vi "S4GUI_003.vi"(7 "Tab ObsEng":enum32{"Obs", "CCD modes", "Guider", "Eng"}(tab)) -> ()   [LabVIEW 2018] (continued)
                n3977 = call-dynamic "Read Channel.vi"("error in (no error)"=w9182, "Acquisition in"=w9181) -> ("error out"=w9184:errorcluster, "Channel.lvclass"=w9183:refnum<class "Channel.lvclass">, "Acquisition out"=w9190:refnum<class "Acquisition.lvclass">)  [unwired: 7 in]
                n3978 = call-dynamic "Read State Machine.vi"("error in (no error)"=w9184, "Device in"=w9183) -> ("error out"=w9186:errorcluster, "State Machine.lvclass"=w9185:refnum<class "State Machine.lvclass">, "Device out"=w9188:refnum<class "Channel.lvclass">)  [unwired: 7 in]
                n3979 = call "Next State.vi"("error in (no error)"=w9186, "New_State"=u32 70, "State Machine in"=w9185) -> ("error out"=w9189:errorcluster, "State Machine out"=w9187:refnum<class "State Machine.lvclass">)  [unwired: 7 in]
                n3980 = call-dynamic "Write State Machine.vi"("error in (no error)"=w9189, "State Machine.lvclass"=w9187, "Device in"=w9188) -> ("error out"=w9191:errorcluster, "Device out"=w9192:refnum<class "Channel.lvclass">)  [unwired: 7 in]
                n3981 = call-dynamic "Write Channel.vi"("error in (no error)"=w9191, "Channel.lvclass"=w9192, "Acquisition in"=w9190) -> ("error out"=w9178:errorcluster, "Acquisition out"=w9179:refnum<class "Acquisition.lvclass">)  [unwired: 7 in]
              }
              frame Enabled {
                # "Não precisa enviar comando STOP para o ACS\nenquanto o controle dos ciclos for feito pela GUI."
              }
            }
            n3982 = call-dynamic "Write Acq_state.vi"("error in (no error)"=w9170, "Acq_state"=u32 0, "Acquisition in"=w9171) -> ("error out"=w9169:errorcluster, "Acquisition out"=w9168:refnum<class "Acquisition.lvclass">)  [unwired: 7 in]
            n3983 = call-dynamic "Write AcquisitionC.vi"("error in (no error)"=w9169, "Acquisition.lvclass"=w9168, "S4ACS_GUI in"=w9174) -> ("error out"=w9156:errorcluster, "S4ACS_GUI out"=w9154:refnum<class "S4GUI.lvclass">)  [unwired: 7 in]
            n3984 = call "Read Instrument.lvclass.vi"("error in (no error)"=w9156, "S4ACS_GUI in"=w9154) -> ("error out"=w9163:errorcluster, "Instrument.lvclass"=w9166:refnum<class "Instrument.lvclass">, "S4ACS_GUI out"=w9167:refnum<class "S4GUI.lvclass">)  [unwired: 7 in]
            n3985 = call "Read WPROT.vi"("error in (no error)"=w9163, "Instrument in"=w9166) -> ("error out"=w9162:errorcluster, "Opt_Selector.lvclass"=w9164:refnum<class "Opt_Selector.lvclass">, "Instrument out"=w9165:refnum<class "Instrument.lvclass">)  [unwired: 7 in]
            n3986 = call-dynamic "Read sequencia_ant.vi"("error in (no error)"=w9162, "Opt_Selector in"=w9164) -> ("error out"=w9158:errorcluster, "sequencia_ant"=w9157:u16, "Opt_Selector out"=w9159:refnum<class "Opt_Selector.lvclass">)  [unwired: 7 in]
            n3987 = call-dynamic "Write sequencia.vi"("error in (no error)"=w9158, "sequencia"=w9157, "Opt_Selector in"=w9159) -> ("error out"=w9145:errorcluster, "Opt_Selector out"=w9148:refnum<class "Opt_Selector.lvclass">)  [unwired: 7 in]
            n3988 = call-dynamic "Read State Machine.vi"("error in (no error)"=w9145, "Device in"=w9148) -> ("error out"=w9150:errorcluster, "State Machine.lvclass"=w9153:refnum<class "State Machine.lvclass">, "Device out"=w9147:refnum<class "Opt_Selector.lvclass">)  [unwired: 7 in]
            n3989 = call "Next State.vi"("error in (no error)"=w9150, "New_State"=10, "State Machine in"=w9153) -> ("error out"=w9149:errorcluster, "State Machine out"=w9152:refnum<class "State Machine.lvclass">)  [unwired: 7 in]
            n3990 = call-dynamic "Write State Machine.vi"("error in (no error)"=w9149, "State Machine.lvclass"=w9152, "Device in"=w9147) -> ("error out"=w9144:errorcluster, "Device out"=w9146:refnum<class "Opt_Selector.lvclass">)  [unwired: 7 in]
            n3991 = call "Write WPROT.vi"("error in (no error)"=w9144, "Opt_Selector.lvclass"=w9146, "Instrument in"=w9165) -> ("error out"=w9161:errorcluster, "Instrument out"=w9160:refnum<class "Instrument.lvclass">)  [unwired: 7 in]
            n3992 = call "Write Instrument.lvclass.vi"("error in (no error)"=w9161, "Instrument.lvclass"=w9160, "S4ACS_GUI in"=w9167) -> ("error out"=w9155:errorcluster, "S4ACS_GUI out"=w9143:refnum<class "S4GUI.lvclass">)  [unwired: 7 in]
          }
          frame Enabled {
            w9200 = FALSE ("Wait Until Done")
            n3993 = call <vilib>:"Application Directory.vi"() -> ("Application Directory"=w9195:path)
            n3994 = Build Path(base path=w9195, name or relative path="MsgStop3.vi") -> (appended path=w9203:path)
            n3995 = Open VI Reference(vi path=w9203, error in (no error)=w9198) -> (vi reference=w9202:refnum<vi>, error out=w9201:errorcluster)  [unwired: 4 in]
            n3996 = invoke class="VI" method="Run VI"(reference=w9202, error in=w9201, "Wait until done"=w9200, "Auto Dispose Ref"=w9200) -> (error out=w9197:errorcluster)  [unwired: 1 in, 4 out]
          }
        }
      }
      event "Stop ch4": Value Change {
        n3997 = event-data() -> ()  [unwired: 1 in, 6 out]
        n3998 = disable-structure shown="Enabled" {
          disable-tunnel: w9207 -> [w9240 w9261]
          disable-tunnel: w9206 -> [w9238 w9263]
          disable-tunnel: [w9220 w9262] -> w9205
          disable-tunnel: [w9208 w9261] -> w9204
          frame Disabled {
            # "Para movimento \nda lamina retardadora"
            # "Restaura a última sequência de lâminas"
            n3999 = call-dynamic "Read AcquisitionD.vi"("error in (no error)"=w9238, "S4ACS_GUI in"=w9240) -> ("error out"=w9242:errorcluster, "Acquisition.lvclass"=w9241:refnum<class "Acquisition.lvclass">, "S4ACS_GUI out"=w9239:refnum<class "S4GUI.lvclass">)  [unwired: 7 in]
            n4000 = disable-structure shown="Enabled" {
              disable-tunnel: w9242 -> [w9247 w9258]
              disable-tunnel: w9241 -> [w9246 w9259]
              disable-tunnel: [w9244 w9259] -> w9236
              disable-tunnel: [w9243 w9258] -> w9235
              frame Disabled {
                # "Só precisa enviar comando STOP quando\no controle dos ciclos for feito pelo ACS."
                n4001 = call-dynamic "Read Channel.vi"("error in (no error)"=w9247, "Acquisition in"=w9246) -> ("error out"=w9249:errorcluster, "Channel.lvclass"=w9248:refnum<class "Channel.lvclass">, "Acquisition out"=w9255:refnum<class "Acquisition.lvclass">)  [unwired: 7 in]
                n4002 = call-dynamic "Read State Machine.vi"("error in (no error)"=w9249, "Device in"=w9248) -> ("error out"=w9251:errorcluster, "State Machine.lvclass"=w9250:refnum<class "State Machine.lvclass">, "Device out"=w9253:refnum<class "Channel.lvclass">)  [unwired: 7 in]
                n4003 = call "Next State.vi"("error in (no error)"=w9251, "New_State"=u32 70, "State Machine in"=w9250) -> ("error out"=w9254:errorcluster, "State Machine out"=w9252:refnum<class "State Machine.lvclass">)  [unwired: 7 in]
                n4004 = call-dynamic "Write State Machine.vi"("error in (no error)"=w9254, "State Machine.lvclass"=w9252, "Device in"=w9253) -> ("error out"=w9256:errorcluster, "Device out"=w9257:refnum<class "Channel.lvclass">)  [unwired: 7 in]
                n4005 = call-dynamic "Write Channel.vi"("error in (no error)"=w9256, "Channel.lvclass"=w9257, "Acquisition in"=w9255) -> ("error out"=w9243:errorcluster, "Acquisition out"=w9244:refnum<class "Acquisition.lvclass">)  [unwired: 7 in]
              }
              frame Enabled {
                # "Não precisa enviar comando STOP para o ACS\nenquanto o controle dos ciclos for feito pela GUI."
              }
            }
            n4006 = call-dynamic "Write Acq_state.vi"("error in (no error)"=w9235, "Acq_state"=u32 0, "Acquisition in"=w9236) -> ("error out"=w9234:errorcluster, "Acquisition out"=w9233:refnum<class "Acquisition.lvclass">)  [unwired: 7 in]
            n4007 = call-dynamic "Write AcquisitionD.vi"("error in (no error)"=w9234, "Acquisition.lvclass"=w9233, "S4ACS_GUI in"=w9239) -> ("error out"=w9221:errorcluster, "S4ACS_GUI out"=w9219:refnum<class "S4GUI.lvclass">)  [unwired: 7 in]
            n4008 = call "Read Instrument.lvclass.vi"("error in (no error)"=w9221, "S4ACS_GUI in"=w9219) -> ("error out"=w9228:errorcluster, "Instrument.lvclass"=w9231:refnum<class "Instrument.lvclass">, "S4ACS_GUI out"=w9232:refnum<class "S4GUI.lvclass">)  [unwired: 7 in]
            n4009 = call "Read WPROT.vi"("error in (no error)"=w9228, "Instrument in"=w9231) -> ("error out"=w9227:errorcluster, "Opt_Selector.lvclass"=w9229:refnum<class "Opt_Selector.lvclass">, "Instrument out"=w9230:refnum<class "Instrument.lvclass">)  [unwired: 7 in]
            n4010 = call-dynamic "Read sequencia_ant.vi"("error in (no error)"=w9227, "Opt_Selector in"=w9229) -> ("error out"=w9223:errorcluster, "sequencia_ant"=w9222:u16, "Opt_Selector out"=w9224:refnum<class "Opt_Selector.lvclass">)  [unwired: 7 in]
            n4011 = call-dynamic "Write sequencia.vi"("error in (no error)"=w9223, "sequencia"=w9222, "Opt_Selector in"=w9224) -> ("error out"=w9210:errorcluster, "Opt_Selector out"=w9213:refnum<class "Opt_Selector.lvclass">)  [unwired: 7 in]
            n4012 = call-dynamic "Read State Machine.vi"("error in (no error)"=w9210, "Device in"=w9213) -> ("error out"=w9215:errorcluster, "State Machine.lvclass"=w9218:refnum<class "State Machine.lvclass">, "Device out"=w9212:refnum<class "Opt_Selector.lvclass">)  [unwired: 7 in]
            n4013 = call "Next State.vi"("error in (no error)"=w9215, "New_State"=10, "State Machine in"=w9218) -> ("error out"=w9214:errorcluster, "State Machine out"=w9217:refnum<class "State Machine.lvclass">)  [unwired: 7 in]
            n4014 = call-dynamic "Write State Machine.vi"("error in (no error)"=w9214, "State Machine.lvclass"=w9217, "Device in"=w9212) -> ("error out"=w9209:errorcluster, "Device out"=w9211:refnum<class "Opt_Selector.lvclass">)  [unwired: 7 in]
            n4015 = call "Write WPROT.vi"("error in (no error)"=w9209, "Opt_Selector.lvclass"=w9211, "Instrument in"=w9230) -> ("error out"=w9226:errorcluster, "Instrument out"=w9225:refnum<class "Instrument.lvclass">)  [unwired: 7 in]
            n4016 = call "Write Instrument.lvclass.vi"("error in (no error)"=w9226, "Instrument.lvclass"=w9225, "S4ACS_GUI in"=w9232) -> ("error out"=w9220:errorcluster, "S4ACS_GUI out"=w9208:refnum<class "S4GUI.lvclass">)  [unwired: 7 in]
          }
          frame Enabled {
            w9265 = FALSE ("Wait Until Done")
            n4017 = call <vilib>:"Application Directory.vi"() -> ("Application Directory"=w9260:path)
            n4018 = Build Path(base path=w9260, name or relative path="MsgStop4.vi") -> (appended path=w9268:path)
            n4019 = Open VI Reference(vi path=w9268, error in (no error)=w9263) -> (vi reference=w9267:refnum<vi>, error out=w9266:errorcluster)  [unwired: 4 in]
            n4020 = invoke class="VI" method="Run VI"(reference=w9267, error in=w9266, "Wait until done"=w9265, "Auto Dispose Ref"=w9265) -> (error out=w9262:errorcluster)  [unwired: 1 in, 4 out]
          }
        }
      }
      event "Pause ch1": Value Change {
        n4021 = event-data() -> ()  [unwired: 1 in, 6 out]
        n4022 = disable-structure shown="Enabled" {
          disable-tunnel: w9272 -> [w9288 w9300]
          disable-tunnel: [w9286 w9298] -> w9271
          disable-tunnel: w9270 -> [w9285 w9299]
          disable-tunnel: [w9273 w9300] -> w9269
          frame Disabled {
            n4023 = call-dynamic "Read AcquisitionA.vi"("error in (no error)"=w9285, "S4ACS_GUI in"=w9288) -> ("error out"=w9280:errorcluster, "Acquisition.lvclass"=w9279:refnum<class "Acquisition.lvclass">, "S4ACS_GUI out"=w9287:refnum<class "S4GUI.lvclass">)  [unwired: 7 in]
            n4024 = call-dynamic "Read Acq_state.vi"("error in (no error)"=w9280, "Acquisition in"=w9279) -> ("error out"=w9282:errorcluster, "Acq_state"=w9283:u32, "Acquisition out"=w9284:refnum<class "Acquisition.lvclass">)  [unwired: 7 in]
            n4025 = call-dynamic "Write Acq_prevstate.vi"("error in (no error)"=w9282, "Acq_prevstate"=w9283, "Acquisition in"=w9284) -> ("error out"=w9277:errorcluster, "Acquisition out"=w9278:refnum<class "Acquisition.lvclass">)  [unwired: 7 in]
            n4026 = call-dynamic "Write Acq_state.vi"("error in (no error)"=w9277, "Acq_state"=u32 400, "Acquisition in"=w9278) -> ("error out"=w9275:errorcluster, "Acquisition out"=w9276:refnum<class "Acquisition.lvclass">)  [unwired: 7 in]
            n4027 = disable-structure shown="Enabled" {
              disable-tunnel: w9275 -> [w9290 w9296]
              disable-tunnel: [w9289 w9296] -> w9274
              frame Disabled {
                n4028 = property on="Start ch1" class="Bool"(error in=w9290, "BoolText.Text"="RESUME" ("Caption.Text")) -> (error out=w9294:errorcluster)  [unwired: 1 in, 1 out]
                n4029 = property on="Pause ch1" class="Bool"(error in=w9294, "DisabledEnum"=T12."Disabled and Grayed Out" ("Disabled")) -> (error out=w9295:errorcluster)  [unwired: 1 in, 1 out]
                n4030 = property on="Start ch1" class="Bool"(error in=w9295, "DisabledEnum"=T12."Enabled" ("Disabled")) -> (error out=w9289:errorcluster)  [unwired: 1 in, 1 out]
              }
              frame Enabled {
              }
            }
            n4031 = call-dynamic "Write AcquisitionA.vi"("error in (no error)"=w9274, "Acquisition.lvclass"=w9276, "S4ACS_GUI in"=w9287) -> ("error out"=w9286:errorcluster, "S4ACS_GUI out"=w9273:refnum<class "S4GUI.lvclass">)  [unwired: 7 in]
          }
          frame Enabled {
            w9302 = FALSE ("Wait Until Done")
            n4032 = call <vilib>:"Application Directory.vi"() -> ("Application Directory"=w9297:path)
            n4033 = Build Path(base path=w9297, name or relative path="MsgPause1.vi") -> (appended path=w9305:path)
            n4034 = Open VI Reference(vi path=w9305, error in (no error)=w9299) -> (vi reference=w9304:refnum<vi>, error out=w9303:errorcluster)  [unwired: 4 in]
            n4035 = invoke class="VI" method="Run VI"(reference=w9304, error in=w9303, "Wait until done"=w9302, "Auto Dispose Ref"=w9302) -> (error out=w9298:errorcluster)  [unwired: 1 in, 4 out]
          }
        }
      }
      event "Pause ch2": Value Change {
        n4036 = event-data() -> ()  [unwired: 1 in, 6 out]
        n4037 = disable-structure shown="Enabled" {
          disable-tunnel: w9309 -> [w9324 w9326]
          disable-tunnel: [w9322 w9327] -> w9308
          disable-tunnel: w9307 -> [w9321 w9328]
          disable-tunnel: [w9311 w9326] -> w9306
          frame Disabled {
            n4038 = call "Read AcquisitionB.vi"("error in (no error)"=w9321, "S4ACS_GUI in"=w9324) -> ("error out"=w9316:errorcluster, "Acquisition.lvclass"=w9315:refnum<class "Acquisition.lvclass">, "S4ACS_GUI out"=w9323:refnum<class "S4GUI.lvclass">)  [unwired: 7 in]
            n4039 = call-dynamic "Read Acq_state.vi"("error in (no error)"=w9316, "Acquisition in"=w9315) -> ("error out"=w9318:errorcluster, "Acq_state"=w9319:u32, "Acquisition out"=w9320:refnum<class "Acquisition.lvclass">)  [unwired: 7 in]
            n4040 = call-dynamic "Write Acq_prevstate.vi"("error in (no error)"=w9318, "Acq_prevstate"=w9319, "Acquisition in"=w9320) -> ("error out"=w9313:errorcluster, "Acquisition out"=w9314:refnum<class "Acquisition.lvclass">)  [unwired: 7 in]
            n4041 = call-dynamic "Write Acq_state.vi"("error in (no error)"=w9313, "Acq_state"=u32 400, "Acquisition in"=w9314) -> ("error out"=w9310:errorcluster, "Acquisition out"=w9312:refnum<class "Acquisition.lvclass">)  [unwired: 7 in]
            n4042 = call "Write AcquisitionB.vi"("error in (no error)"=w9310, "Acquisition.lvclass"=w9312, "S4ACS_GUI in"=w9323) -> ("error out"=w9322:errorcluster, "S4ACS_GUI out"=w9311:refnum<class "S4GUI.lvclass">)  [unwired: 7 in]
          }
          frame Enabled {
            w9330 = FALSE ("Wait Until Done")
            n4043 = call <vilib>:"Application Directory.vi"() -> ("Application Directory"=w9325:path)
            n4044 = Build Path(base path=w9325, name or relative path="MsgPause2.vi") -> (appended path=w9333:path)
            n4045 = Open VI Reference(vi path=w9333, error in (no error)=w9328) -> (vi reference=w9332:refnum<vi>, error out=w9331:errorcluster)  [unwired: 4 in]
            n4046 = invoke class="VI" method="Run VI"(reference=w9332, error in=w9331, "Wait until done"=w9330, "Auto Dispose Ref"=w9330) -> (error out=w9327:errorcluster)  [unwired: 1 in, 4 out]
          }
        }
      }
      event "Pause ch3": Value Change {
        n4047 = event-data() -> ()  [unwired: 1 in, 6 out]
        n4048 = disable-structure shown="Enabled" {
          disable-tunnel: w9337 -> [w9352 w9354]
          disable-tunnel: [w9350 w9355] -> w9336
          disable-tunnel: w9335 -> [w9349 w9356]
          disable-tunnel: [w9339 w9354] -> w9334
          frame Disabled {
            n4049 = call-dynamic "Read AcquisitionC.vi"("error in (no error)"=w9349, "S4ACS_GUI in"=w9352) -> ("error out"=w9344:errorcluster, "Acquisition.lvclass"=w9343:refnum<class "Acquisition.lvclass">, "S4ACS_GUI out"=w9351:refnum<class "S4GUI.lvclass">)  [unwired: 7 in]
            n4050 = call-dynamic "Read Acq_state.vi"("error in (no error)"=w9344, "Acquisition in"=w9343) -> ("error out"=w9346:errorcluster, "Acq_state"=w9347:u32, "Acquisition out"=w9348:refnum<class "Acquisition.lvclass">)  [unwired: 7 in]
            n4051 = call-dynamic "Write Acq_prevstate.vi"("error in (no error)"=w9346, "Acq_prevstate"=w9347, "Acquisition in"=w9348) -> ("error out"=w9341:errorcluster, "Acquisition out"=w9342:refnum<class "Acquisition.lvclass">)  [unwired: 7 in]
            n4052 = call-dynamic "Write Acq_state.vi"("error in (no error)"=w9341, "Acq_state"=u32 400, "Acquisition in"=w9342) -> ("error out"=w9338:errorcluster, "Acquisition out"=w9340:refnum<class "Acquisition.lvclass">)  [unwired: 7 in]
            n4053 = call-dynamic "Write AcquisitionC.vi"("error in (no error)"=w9338, "Acquisition.lvclass"=w9340, "S4ACS_GUI in"=w9351) -> ("error out"=w9350:errorcluster, "S4ACS_GUI out"=w9339:refnum<class "S4GUI.lvclass">)  [unwired: 7 in]
          }
          frame Enabled {
            w9358 = FALSE ("Wait Until Done")
            n4054 = call <vilib>:"Application Directory.vi"() -> ("Application Directory"=w9353:path)
            n4055 = Build Path(base path=w9353, name or relative path="MsgPause3.vi") -> (appended path=w9361:path)
            n4056 = Open VI Reference(vi path=w9361, error in (no error)=w9356) -> (vi reference=w9360:refnum<vi>, error out=w9359:errorcluster)  [unwired: 4 in]
            n4057 = invoke class="VI" method="Run VI"(reference=w9360, error in=w9359, "Wait until done"=w9358, "Auto Dispose Ref"=w9358) -> (error out=w9355:errorcluster)  [unwired: 1 in, 4 out]
          }
        }
      }
      event "Pause ch4": Value Change {
        n4058 = event-data() -> ()  [unwired: 1 in, 6 out]
        n4059 = disable-structure shown="Enabled" {
          disable-tunnel: w9365 -> [w9380 w9389]
          disable-tunnel: [w9378 w9382] -> w9364
          disable-tunnel: w9363 -> [w9377 w9383]
          disable-tunnel: [w9367 w9389] -> w9362
          frame Disabled {
            n4060 = call-dynamic "Read AcquisitionD.vi"("error in (no error)"=w9377, "S4ACS_GUI in"=w9380) -> ("error out"=w9372:errorcluster, "Acquisition.lvclass"=w9371:refnum<class "Acquisition.lvclass">, "S4ACS_GUI out"=w9379:refnum<class "S4GUI.lvclass">)  [unwired: 7 in]
            n4061 = call-dynamic "Read Acq_state.vi"("error in (no error)"=w9372, "Acquisition in"=w9371) -> ("error out"=w9374:errorcluster, "Acq_state"=w9375:u32, "Acquisition out"=w9376:refnum<class "Acquisition.lvclass">)  [unwired: 7 in]
            n4062 = call-dynamic "Write Acq_prevstate.vi"("error in (no error)"=w9374, "Acq_prevstate"=w9375, "Acquisition in"=w9376) -> ("error out"=w9369:errorcluster, "Acquisition out"=w9370:refnum<class "Acquisition.lvclass">)  [unwired: 7 in]
            n4063 = call-dynamic "Write Acq_state.vi"("error in (no error)"=w9369, "Acq_state"=u32 400, "Acquisition in"=w9370) -> ("error out"=w9366:errorcluster, "Acquisition out"=w9368:refnum<class "Acquisition.lvclass">)  [unwired: 7 in]
            n4064 = call-dynamic "Write AcquisitionD.vi"("error in (no error)"=w9366, "Acquisition.lvclass"=w9368, "S4ACS_GUI in"=w9379) -> ("error out"=w9378:errorcluster, "S4ACS_GUI out"=w9367:refnum<class "S4GUI.lvclass">)  [unwired: 7 in]
          }
          frame Enabled {
            w9385 = FALSE ("Wait Until Done")
            n4065 = call <vilib>:"Application Directory.vi"() -> ("Application Directory"=w9381:path)
            n4066 = Build Path(base path=w9381, name or relative path="MsgPause4.vi") -> (appended path=w9388:path)
            n4067 = Open VI Reference(vi path=w9388, error in (no error)=w9383) -> (vi reference=w9387:refnum<vi>, error out=w9386:errorcluster)  [unwired: 4 in]
            n4068 = invoke class="VI" method="Run VI"(reference=w9387, error in=w9386, "Wait until done"=w9385, "Auto Dispose Ref"=w9385) -> (error out=w9382:errorcluster)  [unwired: 1 in, 4 out]
          }
        }
      }
      event "Stop SM": Value Change {
        w9395 = 0.0 ("Scale.Range:Minor Increment")
        n4069 = event-data() -> ()  [unwired: 1 in, 6 out]
        n4070 = call-dynamic "Write User Event.vi"("error in (no error)"=w9393, "User Event"="STOP SM CLICKED", "S4GUI in"=w9394) -> ("error out"=w9391:errorcluster, "S4GUI out"=w9392:refnum<class "S4GUI.lvclass">)  [unwired: 7 in]
        n4071 = disable-structure shown="Enabled" {
          disable-tunnel: w9392 -> [w9432 w9456]
          disable-tunnel: w9391 -> [w9430 w9457]
          disable-tunnel: [w9417 w9455] -> w9397
          disable-tunnel: [w9401 w9456] -> w9396
          frame Disabled {
            # "Não precisa enviar comando STOP para o ACS\nenquanto o controle dos ciclos for feito pela GUI."
            # "Para movimento \nda lamina retardadora"
            # "Restaura a sequencia anterior"
            n4072 = call-dynamic "Read AcquisitionA.vi"("error in (no error)"=w9430, "S4ACS_GUI in"=w9432) -> ("error out"=w9434:errorcluster, "Acquisition.lvclass"=w9433:refnum<class "Acquisition.lvclass">, "S4ACS_GUI out"=w9431:refnum<class "S4GUI.lvclass">)  [unwired: 7 in]
            n4073 = disable-structure shown="Enabled" {
              disable-tunnel: [w9448 w9452] -> w9436
              disable-tunnel: [w9447 w9453] -> w9435
              disable-tunnel: w9434 -> [w9439 w9452]
              disable-tunnel: w9433 -> [w9438 w9453]
              frame Disabled {
                n4074 = call-dynamic "Read Channel.vi"("error in (no error)"=w9439, "Acquisition in"=w9438) -> ("error out"=w9441:errorcluster, "Channel.lvclass"=w9440:refnum<class "Channel.lvclass">, "Acquisition out"=w9449:refnum<class "Acquisition.lvclass">)  [unwired: 7 in]
                n4075 = call-dynamic "Read State Machine.vi"("error in (no error)"=w9441, "Device in"=w9440) -> ("error out"=w9443:errorcluster, "State Machine.lvclass"=w9442:refnum<class "State Machine.lvclass">, "Device out"=w9445:refnum<class "Channel.lvclass">)  [unwired: 7 in]
                n4076 = call "Next State.vi"("error in (no error)"=w9443, "New_State"=u32 70, "State Machine in"=w9442) -> ("error out"=w9446:errorcluster, "State Machine out"=w9444:refnum<class "State Machine.lvclass">)  [unwired: 7 in]
                n4077 = call-dynamic "Write State Machine.vi"("error in (no error)"=w9446, "State Machine.lvclass"=w9444, "Device in"=w9445) -> ("error out"=w9450:errorcluster, "Device out"=w9451:refnum<class "Channel.lvclass">)  [unwired: 7 in]
                n4078 = call-dynamic "Write Channel.vi"("error in (no error)"=w9450, "Channel.lvclass"=w9451, "Acquisition in"=w9449) -> ("error out"=w9448:errorcluster, "Acquisition out"=w9447:refnum<class "Acquisition.lvclass">)  [unwired: 7 in]
              }
              frame Enabled {
              }
            }
            n4079 = call-dynamic "Write AcquisitionA.vi"("error in (no error)"=w9436, "Acquisition.lvclass"=w9435, "S4ACS_GUI in"=w9431) -> ("error out"=w9399:errorcluster, "S4ACS_GUI out"=w9400:refnum<class "S4GUI.lvclass">)  [unwired: 7 in]
            n4080 = call-dynamic "Write Obs_state.vi"("error in (no error)"=w9399, "Obs_state"=u32 0, "S4ACS_GUI in"=w9400) -> ("error out"=w9419:errorcluster, "S4ACS_GUI out"=w9420:refnum<class "S4GUI.lvclass">)  [unwired: 7 in]
            n4081 = call "Read Instrument.lvclass.vi"("error in (no error)"=w9419, "S4ACS_GUI in"=w9420) -> ("error out"=w9428:errorcluster, "Instrument.lvclass"=w9426:refnum<class "Instrument.lvclass">, "S4ACS_GUI out"=w9427:refnum<class "S4GUI.lvclass">)  [unwired: 7 in]
            n4082 = call "Read WPROT.vi"("error in (no error)"=w9428, "Instrument in"=w9426) -> ("error out"=w9413:errorcluster, "Opt_Selector.lvclass"=w9416:refnum<class "Opt_Selector.lvclass">, "Instrument out"=w9425:refnum<class "Instrument.lvclass">)  [unwired: 7 in]
            n4083 = call-dynamic "Read sequencia_ant.vi"("error in (no error)"=w9413, "Opt_Selector in"=w9416) -> ("error out"=w9412:errorcluster, "sequencia_ant"=w9414:u16, "Opt_Selector out"=w9415:refnum<class "Opt_Selector.lvclass">)  [unwired: 7 in]
            n4084 = call-dynamic "Write sequencia.vi"("error in (no error)"=w9412, "sequencia"=w9414, "Opt_Selector in"=w9415) -> ("error out"=w9410:errorcluster, "Opt_Selector out"=w9411:refnum<class "Opt_Selector.lvclass">)  [unwired: 7 in]
            n4085 = call-dynamic "Read State Machine.vi"("error in (no error)"=w9410, "Device in"=w9411) -> ("error out"=w9405:errorcluster, "State Machine.lvclass"=w9408:refnum<class "State Machine.lvclass">, "Device out"=w9409:refnum<class "Opt_Selector.lvclass">)  [unwired: 7 in]
            n4086 = call "Next State.vi"("error in (no error)"=w9405, "New_State"=10, "State Machine in"=w9408) -> ("error out"=w9404:errorcluster, "State Machine out"=w9407:refnum<class "State Machine.lvclass">)  [unwired: 7 in]
            n4087 = call-dynamic "Write State Machine.vi"("error in (no error)"=w9404, "State Machine.lvclass"=w9407, "Device in"=w9409) -> ("error out"=w9403:errorcluster, "Device out"=w9402:refnum<class "Opt_Selector.lvclass">)  [unwired: 7 in]
            n4088 = call "Write WPROT.vi"("error in (no error)"=w9403, "Opt_Selector.lvclass"=w9402, "Instrument in"=w9425) -> ("error out"=w9423:errorcluster, "Instrument out"=w9424:refnum<class "Instrument.lvclass">)  [unwired: 7 in]
            n4089 = call "Write Instrument.lvclass.vi"("error in (no error)"=w9423, "Instrument.lvclass"=w9424, "S4ACS_GUI in"=w9427) -> ("error out"=w9422:errorcluster, "S4ACS_GUI out"=w9421:refnum<class "S4GUI.lvclass">)  [unwired: 7 in]
            n4090 = call-dynamic "Write ciclos.vi"("error in (no error)"=w9422, "ciclos"=u32 0, "S4ACS_GUI in"=w9421) -> ("error out"=w9417:errorcluster, "S4ACS_GUI out"=w9401:refnum<class "S4GUI.lvclass">)  [unwired: 7 in]
          }
          frame Enabled {
            w9459 = FALSE ("Wait Until Done")
            n4091 = call <vilib>:"Application Directory.vi"() -> ("Application Directory"=w9454:path)
            n4092 = Build Path(base path=w9454, name or relative path="MsgStopSync.vi") -> (appended path=w9462:path)
            n4093 = Open VI Reference(vi path=w9462, error in (no error)=w9457) -> (vi reference=w9461:refnum<vi>, error out=w9460:errorcluster)  [unwired: 4 in]
            n4094 = invoke class="VI" method="Run VI"(reference=w9461, error in=w9460, "Wait until done"=w9459, "Auto Dispose Ref"=w9459) -> (error out=w9455:errorcluster)  [unwired: 1 in, 4 out]
          }
        }
        n4095 = property on="#Cycles Done" class="Slide (strict)"(error in=w9397, "Scale.Maximum"=w9395, "Scale.Minimum"=w9395) -> (error out=w9398:errorcluster)  [unwired: 1 in, 1 out]
      }
      event "Abort SM": Value Change {
        w9470 = 0.0 ("Scale.Range:Minor Increment")
        n4096 = event-data() -> ()  [unwired: 1 in, 6 out]
        n4097 = call-dynamic "Write User Event.vi"("error in (no error)"=w9466, "User Event"="ABORT SM CLICKED", "S4GUI in"=w9467) -> ("error out"=w9464:errorcluster, "S4GUI out"=w9465:refnum<class "S4GUI.lvclass">)  [unwired: 7 in]
        n4098 = disable-structure shown="Enabled" {
          disable-tunnel: w9465 -> [w9561 w9585]
          disable-tunnel: w9464 -> [w9559 w9587]
          disable-tunnel: [w9473 w9585] -> w9469
          disable-tunnel: [w9472 w9586] -> w9468
          frame Disabled {
            # "Restaura a sequencia anterior"
            # "Para movimento \nda lamina retardadora"
            n4099 = call-dynamic "Read AcquisitionA.vi"("error in (no error)"=w9559, "S4ACS_GUI in"=w9561) -> ("error out"=w9564:errorcluster, "Acquisition.lvclass"=w9563:refnum<class "Acquisition.lvclass">, "S4ACS_GUI out"=w9560:refnum<class "S4GUI.lvclass">)  [unwired: 7 in]
            n4100 = call-dynamic "Read Channel.vi"("error in (no error)"=w9564, "Acquisition in"=w9563) -> ("error out"=w9566:errorcluster, "Channel.lvclass"=w9565:refnum<class "Channel.lvclass">, "Acquisition out"=w9574:refnum<class "Acquisition.lvclass">)  [unwired: 7 in]
            n4101 = call-dynamic "Read State Machine.vi"("error in (no error)"=w9566, "Device in"=w9565) -> ("error out"=w9568:errorcluster, "State Machine.lvclass"=w9567:refnum<class "State Machine.lvclass">, "Device out"=w9570:refnum<class "Channel.lvclass">)  [unwired: 7 in]
            n4102 = call "Next State.vi"("error in (no error)"=w9568, "New_State"=u32 80, "State Machine in"=w9567) -> ("error out"=w9571:errorcluster, "State Machine out"=w9569:refnum<class "State Machine.lvclass">)  [unwired: 7 in]
            n4103 = call-dynamic "Write State Machine.vi"("error in (no error)"=w9571, "State Machine.lvclass"=w9569, "Device in"=w9570) -> ("error out"=w9575:errorcluster, "Device out"=w9576:refnum<class "Channel.lvclass">)  [unwired: 7 in]
            n4104 = call-dynamic "Write Channel.vi"("error in (no error)"=w9575, "Channel.lvclass"=w9576, "Acquisition in"=w9574) -> ("error out"=w9573:errorcluster, "Acquisition out"=w9572:refnum<class "Acquisition.lvclass">)  [unwired: 7 in]
            n4105 = call-dynamic "Write AcquisitionA.vi"("error in (no error)"=w9573, "Acquisition.lvclass"=w9572, "S4ACS_GUI in"=w9560) -> ("error out"=w9545:errorcluster, "S4ACS_GUI out"=w9544:refnum<class "S4GUI.lvclass">)  [unwired: 7 in]
            n4106 = call "Read AcquisitionB.vi"("error in (no error)"=w9545, "S4ACS_GUI in"=w9544) -> ("error out"=w9538:errorcluster, "Acquisition.lvclass"=w9542:refnum<class "Acquisition.lvclass">, "S4ACS_GUI out"=w9543:refnum<class "S4GUI.lvclass">)  [unwired: 7 in]
            n4107 = call-dynamic "Read Channel.vi"("error in (no error)"=w9538, "Acquisition in"=w9542) -> ("error out"=w9553:errorcluster, "Channel.lvclass"=w9554:refnum<class "Channel.lvclass">, "Acquisition out"=w9540:refnum<class "Acquisition.lvclass">)  [unwired: 7 in]
            n4108 = call-dynamic "Read State Machine.vi"("error in (no error)"=w9553, "Device in"=w9554) -> ("error out"=w9551:errorcluster, "State Machine.lvclass"=w9552:refnum<class "State Machine.lvclass">, "Device out"=w9549:refnum<class "Channel.lvclass">)  [unwired: 7 in]
            n4109 = call "Next State.vi"("error in (no error)"=w9551, "New_State"=u32 80, "State Machine in"=w9552) -> ("error out"=w9548:errorcluster, "State Machine out"=w9550:refnum<class "State Machine.lvclass">)  [unwired: 7 in]
            n4110 = call-dynamic "Write State Machine.vi"("error in (no error)"=w9548, "State Machine.lvclass"=w9550, "Device in"=w9549) -> ("error out"=w9547:errorcluster, "Device out"=w9546:refnum<class "Channel.lvclass">)  [unwired: 7 in]
            n4111 = call-dynamic "Write Channel.vi"("error in (no error)"=w9547, "Channel.lvclass"=w9546, "Acquisition in"=w9540) -> ("error out"=w9539:errorcluster, "Acquisition out"=w9541:refnum<class "Acquisition.lvclass">)  [unwired: 7 in]
            n4112 = call "Write AcquisitionB.vi"("error in (no error)"=w9539, "Acquisition.lvclass"=w9541, "S4ACS_GUI in"=w9543) -> ("error out"=w9505:errorcluster, "S4ACS_GUI out"=w9504:refnum<class "S4GUI.lvclass">)  [unwired: 7 in]
            n4113 = call-dynamic "Read AcquisitionC.vi"("error in (no error)"=w9505, "S4ACS_GUI in"=w9504) -> ("error out"=w9522:errorcluster, "Acquisition.lvclass"=w9526:refnum<class "Acquisition.lvclass">, "S4ACS_GUI out"=w9527:refnum<class "S4GUI.lvclass">)  [unwired: 7 in]
            n4114 = call-dynamic "Read Channel.vi"("error in (no error)"=w9522, "Acquisition in"=w9526) -> ("error out"=w9535:errorcluster, "Channel.lvclass"=w9536:refnum<class "Channel.lvclass">, "Acquisition out"=w9524:refnum<class "Acquisition.lvclass">)  [unwired: 7 in]
            n4115 = call-dynamic "Read State Machine.vi"("error in (no error)"=w9535, "Device in"=w9536) -> ("error out"=w9533:errorcluster, "State Machine.lvclass"=w9534:refnum<class "State Machine.lvclass">, "Device out"=w9531:refnum<class "Channel.lvclass">)  [unwired: 7 in]
            n4116 = call "Next State.vi"("error in (no error)"=w9533, "New_State"=u32 80, "State Machine in"=w9534) -> ("error out"=w9530:errorcluster, "State Machine out"=w9532:refnum<class "State Machine.lvclass">)  [unwired: 7 in]
            n4117 = call-dynamic "Write State Machine.vi"("error in (no error)"=w9530, "State Machine.lvclass"=w9532, "Device in"=w9531) -> ("error out"=w9529:errorcluster, "Device out"=w9528:refnum<class "Channel.lvclass">)  [unwired: 7 in]
            n4118 = call-dynamic "Write Channel.vi"("error in (no error)"=w9529, "Channel.lvclass"=w9528, "Acquisition in"=w9524) -> ("error out"=w9523:errorcluster, "Acquisition out"=w9525:refnum<class "Acquisition.lvclass">)  [unwired: 7 in]
            n4119 = call-dynamic "Write AcquisitionC.vi"("error in (no error)"=w9523, "Acquisition.lvclass"=w9525, "S4ACS_GUI in"=w9527) -> ("error out"=w9503:errorcluster, "S4ACS_GUI out"=w9502:refnum<class "S4GUI.lvclass">)  [unwired: 7 in]
            n4120 = call-dynamic "Read AcquisitionD.vi"("error in (no error)"=w9503, "S4ACS_GUI in"=w9502) -> ("error out"=w9506:errorcluster, "Acquisition.lvclass"=w9510:refnum<class "Acquisition.lvclass">, "S4ACS_GUI out"=w9511:refnum<class "S4GUI.lvclass">)  [unwired: 7 in]
            n4121 = call-dynamic "Read Channel.vi"("error in (no error)"=w9506, "Acquisition in"=w9510) -> ("error out"=w9519:errorcluster, "Channel.lvclass"=w9520:refnum<class "Channel.lvclass">, "Acquisition out"=w9508:refnum<class "Acquisition.lvclass">)  [unwired: 7 in]
            n4122 = call-dynamic "Read State Machine.vi"("error in (no error)"=w9519, "Device in"=w9520) -> ("error out"=w9517:errorcluster, "State Machine.lvclass"=w9518:refnum<class "State Machine.lvclass">, "Device out"=w9515:refnum<class "Channel.lvclass">)  [unwired: 7 in]
            n4123 = call "Next State.vi"("error in (no error)"=w9517, "New_State"=u32 80, "State Machine in"=w9518) -> ("error out"=w9514:errorcluster, "State Machine out"=w9516:refnum<class "State Machine.lvclass">)  [unwired: 7 in]
            n4124 = call-dynamic "Write State Machine.vi"("error in (no error)"=w9514, "State Machine.lvclass"=w9516, "Device in"=w9515) -> ("error out"=w9513:errorcluster, "Device out"=w9512:refnum<class "Channel.lvclass">)  [unwired: 7 in]
            n4125 = call-dynamic "Write Channel.vi"("error in (no error)"=w9513, "Channel.lvclass"=w9512, "Acquisition in"=w9508) -> ("error out"=w9507:errorcluster, "Acquisition out"=w9509:refnum<class "Acquisition.lvclass">)  [unwired: 7 in]
            n4126 = call-dynamic "Write AcquisitionD.vi"("error in (no error)"=w9507, "Acquisition.lvclass"=w9509, "S4ACS_GUI in"=w9511) -> ("error out"=w9500:errorcluster, "S4ACS_GUI out"=w9501:refnum<class "S4GUI.lvclass">)  [unwired: 7 in]
            n4127 = disable-structure shown="Enabled" {
              disable-tunnel: w9501 -> [w9581 w9583]
              disable-tunnel: w9500 -> [w9580 w9582]
              disable-tunnel: [w9578 w9583] -> w9557
              disable-tunnel: [w9577 w9582] -> w9556
              frame Disabled {
                n4128 = call-dynamic "Write aborted.vi"("error in (no error)"=w9580, "aborted"=TRUE ("stopped"), "S4ACS_GUI in"=w9581) -> ("error out"=w9577:errorcluster, "S4ACS_GUI out"=w9578:refnum<class "S4GUI.lvclass">)  [unwired: 7 in]
              }
              frame Enabled {
              }
            }
            n4129 = call-dynamic "Write Obs_state.vi"("error in (no error)"=w9556, "Obs_state"=u32 0, "S4ACS_GUI in"=w9557) -> ("error out"=w9474:errorcluster, "S4ACS_GUI out"=w9475:refnum<class "S4GUI.lvclass">)  [unwired: 7 in]
            n4130 = call "Read Instrument.lvclass.vi"("error in (no error)"=w9474, "S4ACS_GUI in"=w9475) -> ("error out"=w9494:errorcluster, "Instrument.lvclass"=w9496:refnum<class "Instrument.lvclass">, "S4ACS_GUI out"=w9495:refnum<class "S4GUI.lvclass">)  [unwired: 7 in]
            n4131 = call "Read WPROT.vi"("error in (no error)"=w9494, "Instrument in"=w9496) -> ("error out"=w9489:errorcluster, "Opt_Selector.lvclass"=w9492:refnum<class "Opt_Selector.lvclass">, "Instrument out"=w9497:refnum<class "Instrument.lvclass">)  [unwired: 7 in]
            n4132 = call-dynamic "Read sequencia_ant.vi"("error in (no error)"=w9489, "Opt_Selector in"=w9492) -> ("error out"=w9488:errorcluster, "sequencia_ant"=w9490:u16, "Opt_Selector out"=w9491:refnum<class "Opt_Selector.lvclass">)  [unwired: 7 in]
            n4133 = call-dynamic "Write sequencia.vi"("error in (no error)"=w9488, "sequencia"=w9490, "Opt_Selector in"=w9491) -> ("error out"=w9483:errorcluster, "Opt_Selector out"=w9484:refnum<class "Opt_Selector.lvclass">)  [unwired: 7 in]
            n4134 = call-dynamic "Read State Machine.vi"("error in (no error)"=w9483, "Device in"=w9484) -> ("error out"=w9486:errorcluster, "State Machine.lvclass"=w9481:refnum<class "State Machine.lvclass">, "Device out"=w9482:refnum<class "Opt_Selector.lvclass">)  [unwired: 7 in]
            n4135 = call "Next State.vi"("error in (no error)"=w9486, "New_State"=10, "State Machine in"=w9481) -> ("error out"=w9485:errorcluster, "State Machine out"=w9480:refnum<class "State Machine.lvclass">)  [unwired: 7 in]
            n4136 = call-dynamic "Write State Machine.vi"("error in (no error)"=w9485, "State Machine.lvclass"=w9480, "Device in"=w9482) -> ("error out"=w9479:errorcluster, "Device out"=w9478:refnum<class "Opt_Selector.lvclass">)  [unwired: 7 in]
            n4137 = call "Write WPROT.vi"("error in (no error)"=w9479, "Opt_Selector.lvclass"=w9478, "Instrument in"=w9497) -> ("error out"=w9476:errorcluster, "Instrument out"=w9477:refnum<class "Instrument.lvclass">)  [unwired: 7 in]
            n4138 = call "Write Instrument.lvclass.vi"("error in (no error)"=w9476, "Instrument.lvclass"=w9477, "S4ACS_GUI in"=w9495) -> ("error out"=w9498:errorcluster, "S4ACS_GUI out"=w9499:refnum<class "S4GUI.lvclass">)  [unwired: 7 in]
            n4139 = call-dynamic "Write ciclos.vi"("error in (no error)"=w9498, "ciclos"=u32 0, "S4ACS_GUI in"=w9499) -> ("error out"=w9472:errorcluster, "S4ACS_GUI out"=w9473:refnum<class "S4GUI.lvclass">)  [unwired: 7 in]
          }
          frame Enabled {
            w9589 = FALSE ("Wait Until Done")
            n4140 = call <vilib>:"Application Directory.vi"() -> ("Application Directory"=w9584:path)
            n4141 = Build Path(base path=w9584, name or relative path="MsgAbortSync.vi") -> (appended path=w9592:path)
            n4142 = Open VI Reference(vi path=w9592, error in (no error)=w9587) -> (vi reference=w9591:refnum<vi>, error out=w9590:errorcluster)  [unwired: 4 in]
            n4143 = invoke class="VI" method="Run VI"(reference=w9591, error in=w9590, "Wait until done"=w9589, "Auto Dispose Ref"=w9589) -> (error out=w9586:errorcluster)  [unwired: 1 in, 4 out]
          }
        }
        n4144 = property on="#Cycles Done" class="Slide (strict)"(error in=w9468, "Scale.Maximum"=w9470, "Scale.Minimum"=w9470) -> (error out=w9471:errorcluster)  [unwired: 1 in, 1 out]
      }
      event "Pause SM": Value Change {
        n4145 = event-data() -> ()  [unwired: 1 in, 6 out]
        n4146 = call-dynamic "Write User Event.vi"("error in (no error)"=w9596, "User Event"="PAUSE SM CLICKED", "S4GUI in"=w9597) -> ("error out"=w9594:errorcluster, "S4GUI out"=w9595:refnum<class "S4GUI.lvclass">)  [unwired: 7 in]
        n4147 = disable-structure shown="Enabled" {
          disable-tunnel: w9595 -> [w9611 w9621]
          disable-tunnel: w9594 -> [w9610 w9622]
          disable-tunnel: [w9601 w9621] -> w9599
          disable-tunnel: [w9600 w9620] -> w9598
          frame Disabled {
            n4148 = disable-structure shown="Enabled" {
              disable-tunnel: w9611 -> [w9615 w9618]
              disable-tunnel: w9610 -> [w9614 w9617]
              disable-tunnel: [w9613 w9618] -> w9604
              disable-tunnel: [w9612 w9617] -> w9603
              frame Disabled {
                n4149 = call-dynamic "Write paused.vi"("error in (no error)"=w9614, "paused"=TRUE ("stopped"), "S4ACS_GUI in"=w9615) -> ("error out"=w9612:errorcluster, "S4ACS_GUI out"=w9613:refnum<class "S4GUI.lvclass">)  [unwired: 7 in]
              }
              frame Enabled {
              }
            }
            n4150 = call-dynamic "Read Obs_state.vi"("error in (no error)"=w9603, "S4ACS_GUI in"=w9604) -> ("error out"=w9607:errorcluster, "Obs_state"=w9609:u32, "S4ACS_GUI out"=w9608:refnum<class "S4GUI.lvclass">)  [unwired: 7 in]
            n4151 = call-dynamic "Write Obs_prevstate.vi"("error in (no error)"=w9607, "Obs_prevstate"=w9609, "S4ACS_GUI in"=w9608) -> ("error out"=w9605:errorcluster, "S4ACS_GUI out"=w9606:refnum<class "S4GUI.lvclass">)  [unwired: 7 in]
            n4152 = call-dynamic "Write Obs_state.vi"("error in (no error)"=w9605, "Obs_state"=u32 400, "S4ACS_GUI in"=w9606) -> ("error out"=w9600:errorcluster, "S4ACS_GUI out"=w9601:refnum<class "S4GUI.lvclass">)  [unwired: 7 in]
          }
          frame Enabled {
            w9624 = FALSE ("Wait Until Done")
            n4153 = call <vilib>:"Application Directory.vi"() -> ("Application Directory"=w9619:path)
            n4154 = Build Path(base path=w9619, name or relative path="MsgPauseSync.vi") -> (appended path=w9627:path)
            n4155 = Open VI Reference(vi path=w9627, error in (no error)=w9622) -> (vi reference=w9626:refnum<vi>, error out=w9625:errorcluster)  [unwired: 4 in]
            n4156 = invoke class="VI" method="Run VI"(reference=w9626, error in=w9625, "Wait until done"=w9624, "Auto Dispose Ref"=w9624) -> (error out=w9620:errorcluster)  [unwired: 1 in, 4 out]
          }
        }
      }
      event "Abort ch1": Value Change {
        n4157 = event-data() -> ()  [unwired: 1 in, 6 out]
        n4158 = disable-structure shown="Enabled" {
          disable-tunnel: w9631 -> [w9664 w9686]
          disable-tunnel: w9630 -> [w9662 w9680]
          disable-tunnel: [w9644 w9679] -> w9629
          disable-tunnel: [w9632 w9686] -> w9628
          frame Disabled {
            # "Para movimento \nda lamina retardadora"
            # "Restaura a última sequência de lâminas"
            n4159 = call-dynamic "Read AcquisitionA.vi"("error in (no error)"=w9662, "S4ACS_GUI in"=w9664) -> ("error out"=w9667:errorcluster, "Acquisition.lvclass"=w9666:refnum<class "Acquisition.lvclass">, "S4ACS_GUI out"=w9663:refnum<class "S4GUI.lvclass">)  [unwired: 7 in]
            n4160 = call-dynamic "Read Channel.vi"("error in (no error)"=w9667, "Acquisition in"=w9666) -> ("error out"=w9669:errorcluster, "Channel.lvclass"=w9668:refnum<class "Channel.lvclass">, "Acquisition out"=w9675:refnum<class "Acquisition.lvclass">)  [unwired: 7 in]
            n4161 = call-dynamic "Read State Machine.vi"("error in (no error)"=w9669, "Device in"=w9668) -> ("error out"=w9671:errorcluster, "State Machine.lvclass"=w9670:refnum<class "State Machine.lvclass">, "Device out"=w9673:refnum<class "Channel.lvclass">)  [unwired: 7 in]
            n4162 = call "Next State.vi"("error in (no error)"=w9671, "New_State"=u32 80, "State Machine in"=w9670) -> ("error out"=w9674:errorcluster, "State Machine out"=w9672:refnum<class "State Machine.lvclass">)  [unwired: 7 in]
            n4163 = call-dynamic "Write State Machine.vi"("error in (no error)"=w9674, "State Machine.lvclass"=w9672, "Device in"=w9673) -> ("error out"=w9676:errorcluster, "Device out"=w9677:refnum<class "Channel.lvclass">)  [unwired: 7 in]
            n4164 = call-dynamic "Write Channel.vi"("error in (no error)"=w9676, "Channel.lvclass"=w9677, "Acquisition in"=w9675) -> ("error out"=w9659:errorcluster, "Acquisition out"=w9660:refnum<class "Acquisition.lvclass">)  [unwired: 7 in]
            n4165 = call-dynamic "Write Acq_state.vi"("error in (no error)"=w9659, "Acq_state"=u32 0, "Acquisition in"=w9660) -> ("error out"=w9658:errorcluster, "Acquisition out"=w9657:refnum<class "Acquisition.lvclass">)  [unwired: 7 in]
            n4166 = call-dynamic "Write AcquisitionA.vi"("error in (no error)"=w9658, "Acquisition.lvclass"=w9657, "S4ACS_GUI in"=w9663) -> ("error out"=w9645:errorcluster, "S4ACS_GUI out"=w9643:refnum<class "S4GUI.lvclass">)  [unwired: 7 in]
            n4167 = call "Read Instrument.lvclass.vi"("error in (no error)"=w9645, "S4ACS_GUI in"=w9643) -> ("error out"=w9652:errorcluster, "Instrument.lvclass"=w9655:refnum<class "Instrument.lvclass">, "S4ACS_GUI out"=w9656:refnum<class "S4GUI.lvclass">)  [unwired: 7 in]
            n4168 = call "Read WPROT.vi"("error in (no error)"=w9652, "Instrument in"=w9655) -> ("error out"=w9651:errorcluster, "Opt_Selector.lvclass"=w9653:refnum<class "Opt_Selector.lvclass">, "Instrument out"=w9654:refnum<class "Instrument.lvclass">)  [unwired: 7 in]
            n4169 = call-dynamic "Read sequencia_ant.vi"("error in (no error)"=w9651, "Opt_Selector in"=w9653) -> ("error out"=w9647:errorcluster, "sequencia_ant"=w9646:u16, "Opt_Selector out"=w9648:refnum<class "Opt_Selector.lvclass">)  [unwired: 7 in]
            n4170 = call-dynamic "Write sequencia.vi"("error in (no error)"=w9647, "sequencia"=w9646, "Opt_Selector in"=w9648) -> ("error out"=w9636:errorcluster, "Opt_Selector out"=w9637:refnum<class "Opt_Selector.lvclass">)  [unwired: 7 in]
            n4171 = call-dynamic "Read State Machine.vi"("error in (no error)"=w9636, "Device in"=w9637) -> ("error out"=w9639:errorcluster, "State Machine.lvclass"=w9642:refnum<class "State Machine.lvclass">, "Device out"=w9635:refnum<class "Opt_Selector.lvclass">)  [unwired: 7 in]
            n4172 = call "Next State.vi"("error in (no error)"=w9639, "New_State"=10, "State Machine in"=w9642) -> ("error out"=w9638:errorcluster, "State Machine out"=w9641:refnum<class "State Machine.lvclass">)  [unwired: 7 in]
            n4173 = call-dynamic "Write State Machine.vi"("error in (no error)"=w9638, "State Machine.lvclass"=w9641, "Device in"=w9635) -> ("error out"=w9633:errorcluster, "Device out"=w9634:refnum<class "Opt_Selector.lvclass">)  [unwired: 7 in]
            n4174 = call "Write WPROT.vi"("error in (no error)"=w9633, "Opt_Selector.lvclass"=w9634, "Instrument in"=w9654) -> ("error out"=w9650:errorcluster, "Instrument out"=w9649:refnum<class "Instrument.lvclass">)  [unwired: 7 in]
            n4175 = call "Write Instrument.lvclass.vi"("error in (no error)"=w9650, "Instrument.lvclass"=w9649, "S4ACS_GUI in"=w9656) -> ("error out"=w9644:errorcluster, "S4ACS_GUI out"=w9632:refnum<class "S4GUI.lvclass">)  [unwired: 7 in]
          }
          frame Enabled {
            w9682 = FALSE ("Wait Until Done")
            n4176 = call <vilib>:"Application Directory.vi"() -> ("Application Directory"=w9678:path)
            n4177 = Build Path(base path=w9678, name or relative path="MsgAbort1.vi") -> (appended path=w9685:path)
            n4178 = Open VI Reference(vi path=w9685, error in (no error)=w9680) -> (vi reference=w9684:refnum<vi>, error out=w9683:errorcluster)  [unwired: 4 in]
            n4179 = invoke class="VI" method="Run VI"(reference=w9684, error in=w9683, "Wait until done"=w9682, "Auto Dispose Ref"=w9682) -> (error out=w9679:errorcluster)  [unwired: 1 in, 4 out]
          }
        }
      }
      event "Abort ch2": Value Change {
        n4180 = event-data() -> ()  [unwired: 1 in, 6 out]
        n4181 = disable-structure shown="Enabled" {
          disable-tunnel: w9690 -> [w9723 w9739]
          disable-tunnel: w9689 -> [w9721 w9740]
          disable-tunnel: [w9703 w9738] -> w9688
          disable-tunnel: [w9691 w9739] -> w9687
          frame Disabled {
            # "Para movimento \nda lamina retardadora"
            # "Restaura a última sequência de lâminas"
            n4182 = call "Read AcquisitionB.vi"("error in (no error)"=w9721, "S4ACS_GUI in"=w9723) -> ("error out"=w9726:errorcluster, "Acquisition.lvclass"=w9725:refnum<class "Acquisition.lvclass">, "S4ACS_GUI out"=w9722:refnum<class "S4GUI.lvclass">)  [unwired: 7 in]
            n4183 = call-dynamic "Read Channel.vi"("error in (no error)"=w9726, "Acquisition in"=w9725) -> ("error out"=w9728:errorcluster, "Channel.lvclass"=w9727:refnum<class "Channel.lvclass">, "Acquisition out"=w9734:refnum<class "Acquisition.lvclass">)  [unwired: 7 in]
            n4184 = call-dynamic "Read State Machine.vi"("error in (no error)"=w9728, "Device in"=w9727) -> ("error out"=w9730:errorcluster, "State Machine.lvclass"=w9729:refnum<class "State Machine.lvclass">, "Device out"=w9732:refnum<class "Channel.lvclass">)  [unwired: 7 in]
            n4185 = call "Next State.vi"("error in (no error)"=w9730, "New_State"=u32 80, "State Machine in"=w9729) -> ("error out"=w9733:errorcluster, "State Machine out"=w9731:refnum<class "State Machine.lvclass">)  [unwired: 7 in]
            n4186 = call-dynamic "Write State Machine.vi"("error in (no error)"=w9733, "State Machine.lvclass"=w9731, "Device in"=w9732) -> ("error out"=w9735:errorcluster, "Device out"=w9736:refnum<class "Channel.lvclass">)  [unwired: 7 in]
            n4187 = call-dynamic "Write Channel.vi"("error in (no error)"=w9735, "Channel.lvclass"=w9736, "Acquisition in"=w9734) -> ("error out"=w9718:errorcluster, "Acquisition out"=w9719:refnum<class "Acquisition.lvclass">)  [unwired: 7 in]
            n4188 = call-dynamic "Write Acq_state.vi"("error in (no error)"=w9718, "Acq_state"=u32 0, "Acquisition in"=w9719) -> ("error out"=w9717:errorcluster, "Acquisition out"=w9716:refnum<class "Acquisition.lvclass">)  [unwired: 7 in]
            n4189 = call "Write AcquisitionB.vi"("error in (no error)"=w9717, "Acquisition.lvclass"=w9716, "S4ACS_GUI in"=w9722) -> ("error out"=w9704:errorcluster, "S4ACS_GUI out"=w9702:refnum<class "S4GUI.lvclass">)  [unwired: 7 in]
            n4190 = call "Read Instrument.lvclass.vi"("error in (no error)"=w9704, "S4ACS_GUI in"=w9702) -> ("error out"=w9711:errorcluster, "Instrument.lvclass"=w9714:refnum<class "Instrument.lvclass">, "S4ACS_GUI out"=w9715:refnum<class "S4GUI.lvclass">)  [unwired: 7 in]
            n4191 = call "Read WPROT.vi"("error in (no error)"=w9711, "Instrument in"=w9714) -> ("error out"=w9710:errorcluster, "Opt_Selector.lvclass"=w9712:refnum<class "Opt_Selector.lvclass">, "Instrument out"=w9713:refnum<class "Instrument.lvclass">)  [unwired: 7 in]
            n4192 = call-dynamic "Read sequencia_ant.vi"("error in (no error)"=w9710, "Opt_Selector in"=w9712) -> ("error out"=w9706:errorcluster, "sequencia_ant"=w9705:u16, "Opt_Selector out"=w9707:refnum<class "Opt_Selector.lvclass">)  [unwired: 7 in]
            n4193 = call-dynamic "Write sequencia.vi"("error in (no error)"=w9706, "sequencia"=w9705, "Opt_Selector in"=w9707) -> ("error out"=w9695:errorcluster, "Opt_Selector out"=w9696:refnum<class "Opt_Selector.lvclass">)  [unwired: 7 in]
            n4194 = call-dynamic "Read State Machine.vi"("error in (no error)"=w9695, "Device in"=w9696) -> ("error out"=w9698:errorcluster, "State Machine.lvclass"=w9701:refnum<class "State Machine.lvclass">, "Device out"=w9694:refnum<class "Opt_Selector.lvclass">)  [unwired: 7 in]
            n4195 = call "Next State.vi"("error in (no error)"=w9698, "New_State"=10, "State Machine in"=w9701) -> ("error out"=w9697:errorcluster, "State Machine out"=w9700:refnum<class "State Machine.lvclass">)  [unwired: 7 in]
            n4196 = call-dynamic "Write State Machine.vi"("error in (no error)"=w9697, "State Machine.lvclass"=w9700, "Device in"=w9694) -> ("error out"=w9692:errorcluster, "Device out"=w9693:refnum<class "Opt_Selector.lvclass">)  [unwired: 7 in]
